vi "Encoder.vi"(1 "Terms":i32, 2 "Timestep":dbl) -> ()   [LabVIEW 2017]
uses:
  Robot Global Data.vi
panel:
  out "Velocity":cluster{dbl, dbl}(graph)
  out "Position":cluster{dbl, dbl}(graph)
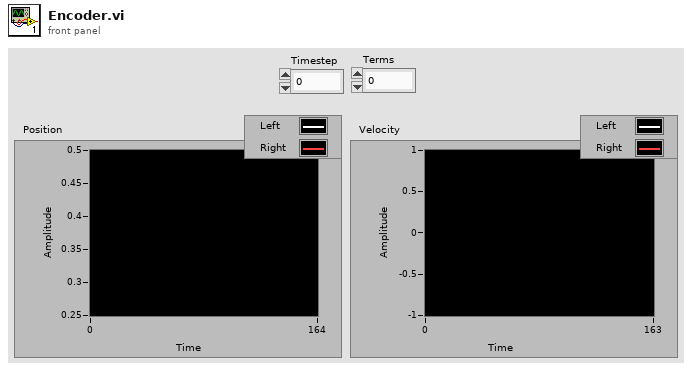
[diagram p1: front panel]
types:
  T1 = typedef "WPI_EncoderDevRef.ctl" = cluster{"DevStatus":errorcluster, "EncoderIndex":T2, "CounterIndex":T3, "DistancePerCount":dbl, "Decoding Type":T4}
  T2 = typedef "FPGA_EncoderIdx.ctl" = enum8{"Enc 0", "Enc 1", "Enc 2", "Enc 3", "Enc 4", "Enc 5", "Enc 6", "Enc 7", "Invalid"}
  T3 = typedef "FPGA_CounterCtrSystemIndex.ctl" = enum8{"Ctr 0", "Ctr 1", "Ctr 2", "Ctr 3", "Ctr 4", "Ctr 5", "Ctr 6", "Ctr 7", "Invalid"}
  T4 = typedef "WPI_EncoderType.ctl" = enum16{"1x", "2x", "4x"}
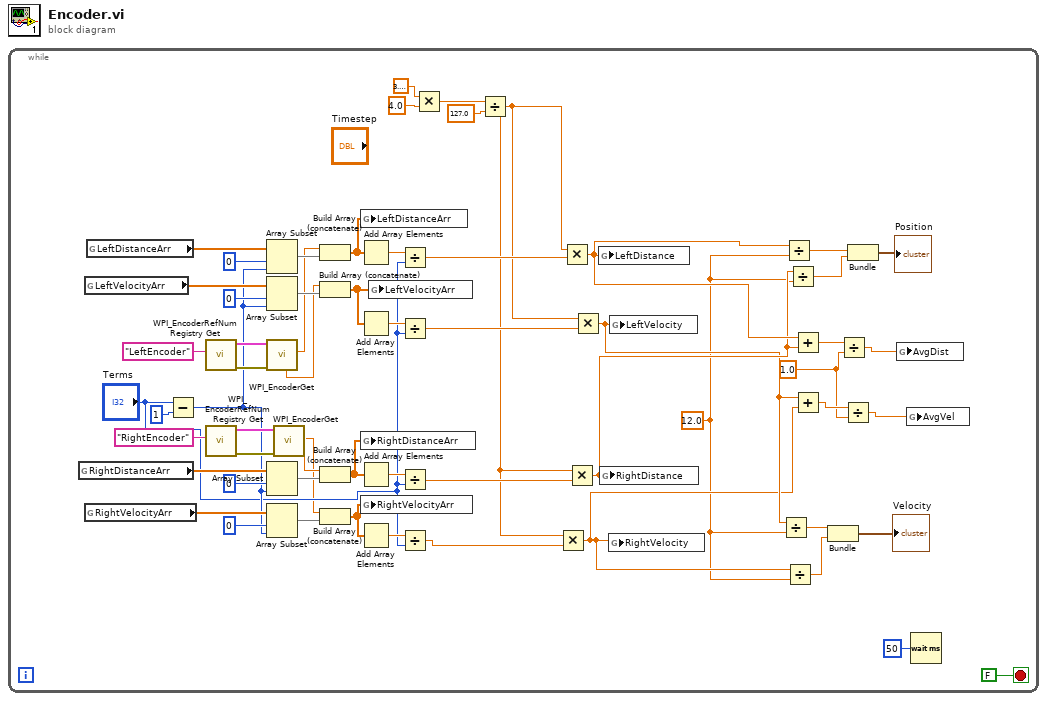
[diagram p0: block diagram]
diagram:
  n1 = while {
    stop <- FALSE stop-if-true
    w3 = 12.0
    w14 = 1.0
    n2 = global read "Robot Global Data.vi" "RightDistanceArr"() -> (w47:dbl[])
    n3 = global read "Robot Global Data.vi" "LeftVelocityArr"() -> (w49:dbl[])
    n4 = global read "Robot Global Data.vi" "RightVelocityArr"() -> (w54:dbl[])
    n5 = global read "Robot Global Data.vi" "LeftDistanceArr"() -> (w51:dbl[])
    n6 = Subtract(x="Terms", y=1) -> (x-y=w43:i32)
    n7 = call <vilib>:"WPI_EncoderRefNum Registry Get.vi"("refnum name"="LeftEncoder") -> ("error out"=w59:errorcluster, "EncoderDevRef"=w60:T1)  [unwired: 9 in]
    n8 = call <vilib>:"WPI_EncoderRefNum Registry Get.vi"("refnum name"="RightEncoder") -> ("error out"=w57:errorcluster, "EncoderDevRef"=w58:T1)  [unwired: 9 in]
    n9 = Array Subset(array=w51, index=0, length=w43) -> (w46:dbl[])
    n10 = Array Subset(array=w49, index=0, length=w43) -> (w42:dbl[])
    n11 = call <vilib>:"WPI_EncoderGet.vi"("error in (no error)"=w59, "EncoderDevRef"=w60) -> ("Distance"=w32:dbl, "Rate"=w31:dbl)  [unwired: 4 in, 4 out]
    n12 = Array Subset(array=w47, index=0, length=w43) -> (w41:dbl[])
    n13 = Array Subset(array=w54, index=0, length=w43) -> (w52:dbl[])
    n14 = call <vilib>:"WPI_EncoderGet.vi"("error in (no error)"=w57, "EncoderDevRef"=w58) -> ("Distance"=w30:dbl, "Rate"=w29:dbl)  [unwired: 4 in, 4 out]
    n15 = Build Array (concatenate)(w32, w46) -> (w39:dbl[])
    n16 = Build Array (concatenate)(w31, w42) -> (w38:dbl[])
    n17 = Build Array (concatenate)(w30, w41) -> (w28:dbl[])
    n18 = Build Array (concatenate)(w29, w52) -> (w40:dbl[])
    n19 = global write "Robot Global Data.vi" "LeftDistanceArr"(w39) -> ()
    n20 = Add Array Elements(numeric array=w39) -> (sum=w36:dbl)
    n21 = Add Array Elements(numeric array=w38) -> (sum=w35:dbl)
    n22 = global write "Robot Global Data.vi" "RightDistanceArr"(w28) -> ()
    n23 = Add Array Elements(numeric array=w28) -> (sum=w34:dbl)
    n24 = global write "Robot Global Data.vi" "RightVelocityArr"(w40) -> ()
    n25 = Add Array Elements(numeric array=w40) -> (sum=w37:dbl)
    n26 = global write "Robot Global Data.vi" "LeftVelocityArr"(w38) -> ()
    n27 = Divide(x=w36, y="Terms") -> (x/y=w23:dbl)
    n28 = Divide(x=w35, y="Terms") -> (x/y=w22:dbl)
    n29 = Divide(x=w34, y="Terms") -> (x/y=w21:dbl)
    n30 = Divide(x=w37, y="Terms") -> (x/y=w19:dbl)
    n31 = Multiply(x=3.141592653589793, y=4.0) -> (x*y=w25:dbl)
    n32 = Divide(x=w25, y=127.0) -> (x/y=w20:dbl)
    n33 = Multiply(x=w20, y=w19) -> (x*y=w4:dbl)
    n34 = Multiply(x=w20, y=w23) -> (x*y=w7:dbl)
    n35 = Multiply(x=w20, y=w21) -> (x*y=w6:dbl)
    n36 = Multiply(x=w20, y=w22) -> (x*y=w5:dbl)
    n37 = global write "Robot Global Data.vi" "LeftDistance"(w7) -> ()
    n38 = global write "Robot Global Data.vi" "RightDistance"(w6) -> ()
    n39 = global write "Robot Global Data.vi" "RightVelocity"(w4) -> ()
    n40 = global write "Robot Global Data.vi" "LeftVelocity"(w5) -> ()
    n41 = Divide(x=w5, y=w3) -> (x/y=w11:dbl)
    n42 = Divide(x=w7, y=w3) -> (x/y=w9:dbl)
    n43 = Divide(x=w4, y=w3) -> (x/y=w10:dbl)
    n44 = Divide(x=w6, y=w3) -> (x/y=w8:dbl)
    n45 = Add(x=w7, y=w6) -> (x+y=w16:dbl)
    n46 = Add(x=w5, y=w4) -> (x+y=w15:dbl)
    n47 = Bundle(w11, w10) -> (→"Velocity":cluster{dbl, dbl})  [unwired: 1 in]
    n48 = Divide(x=w16, y=w14) -> (x/y=w13:dbl)
    n49 = Divide(x=w15, y=w14) -> (x/y=w12:dbl)
    n50 = Bundle(w9, w8) -> (→"Position":cluster{dbl, dbl})  [unwired: 1 in]
    n51 = global write "Robot Global Data.vi" "AvgDist"(w13) -> ()
    n52 = global write "Robot Global Data.vi" "AvgVel"(w12) -> ()
    n53 = Wait (ms)(milliseconds to wait=u32 50) -> ()  [unwired: 1 out]
  }
